vi "Auto_guider_queued.vi"() -> ()   [LabVIEW 2018]
uses:
  Global_Telescopio.vi
panel:
  out "respQ":refnum<queue>
  out "cmdQ":refnum<queue>
  in  "Case Constant\n(See Context Help) 2":bool
  in  "Case Constant\n(See Context Help)":bool=TRUE
  out "substring 3":string
  out "substring 2":string
  out "concatenated string":string
  out "substring":string
  out "result string":string
  in  "esc_placa":string="0.462"
  in  "guide_esp":string="S"
  in  "guide_cas":string="S"
  in  "guide_str":string="04/10/09  1:18:34\u000013 27 13\u0000-12 45 20\u0000"
  in  "guide_ang":string=" 281.52"
  in  "guide_nor":string="  11.53"
  in  "Tx_sts":u8[](array[numeric])=[22, 2, 1, 0, 83, 0, 0]
  out "rxsts 3":bool
  in  "SYN | ETX":u8[](array[numeric])=[22, 3] format="%02.0f"
  in  "tel_sts2":u8[](array[numeric])=[0, 0, 0] format="%02.0f"
  in  "Tx_ena":u8[](array[numeric])=[22, 2, 1, 0, 72, 0, 0] format="%02.0f"
  out "tel_sts1":bool[](array[boolean])=[TRUE, TRUE, TRUE, TRUE, FALSE, FALSE, TRUE]
  out "guide_dec":dbl format="%07.2g"
  out "guide_dir_ns":string
  out "guide_asc":dbl format="%07.2g"
  out "guide_dir_we":string
  in  "SYN | ACK":u8[](array[numeric])=[22, 6] format="%02.0f"
  out "rxsts":bool
  in  "Tx_nak":u8[](array[numeric])=[22, 21]
  out "Data rx guider":string
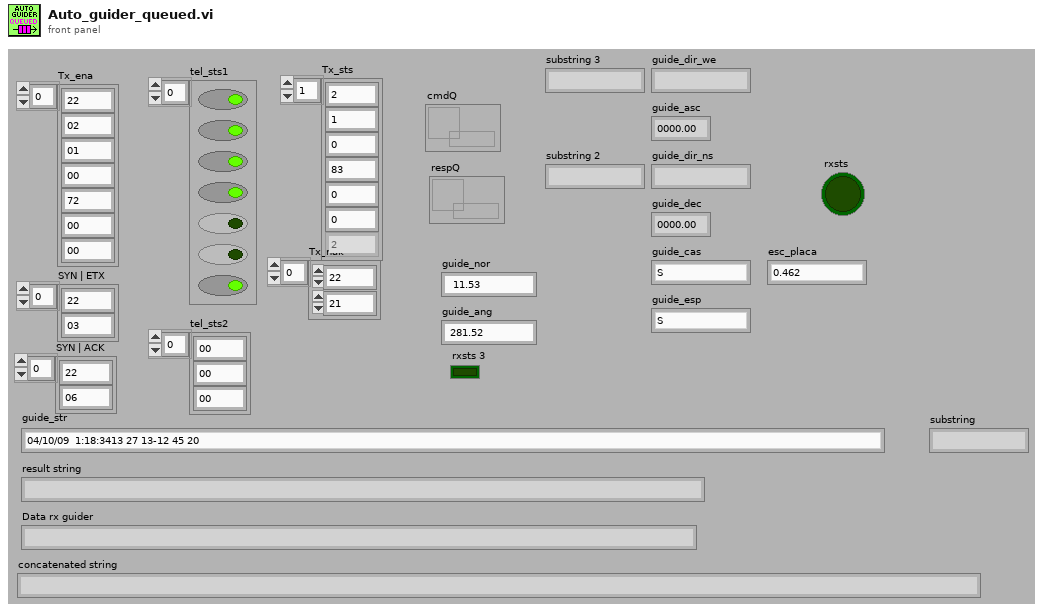
[diagram p1: front panel]
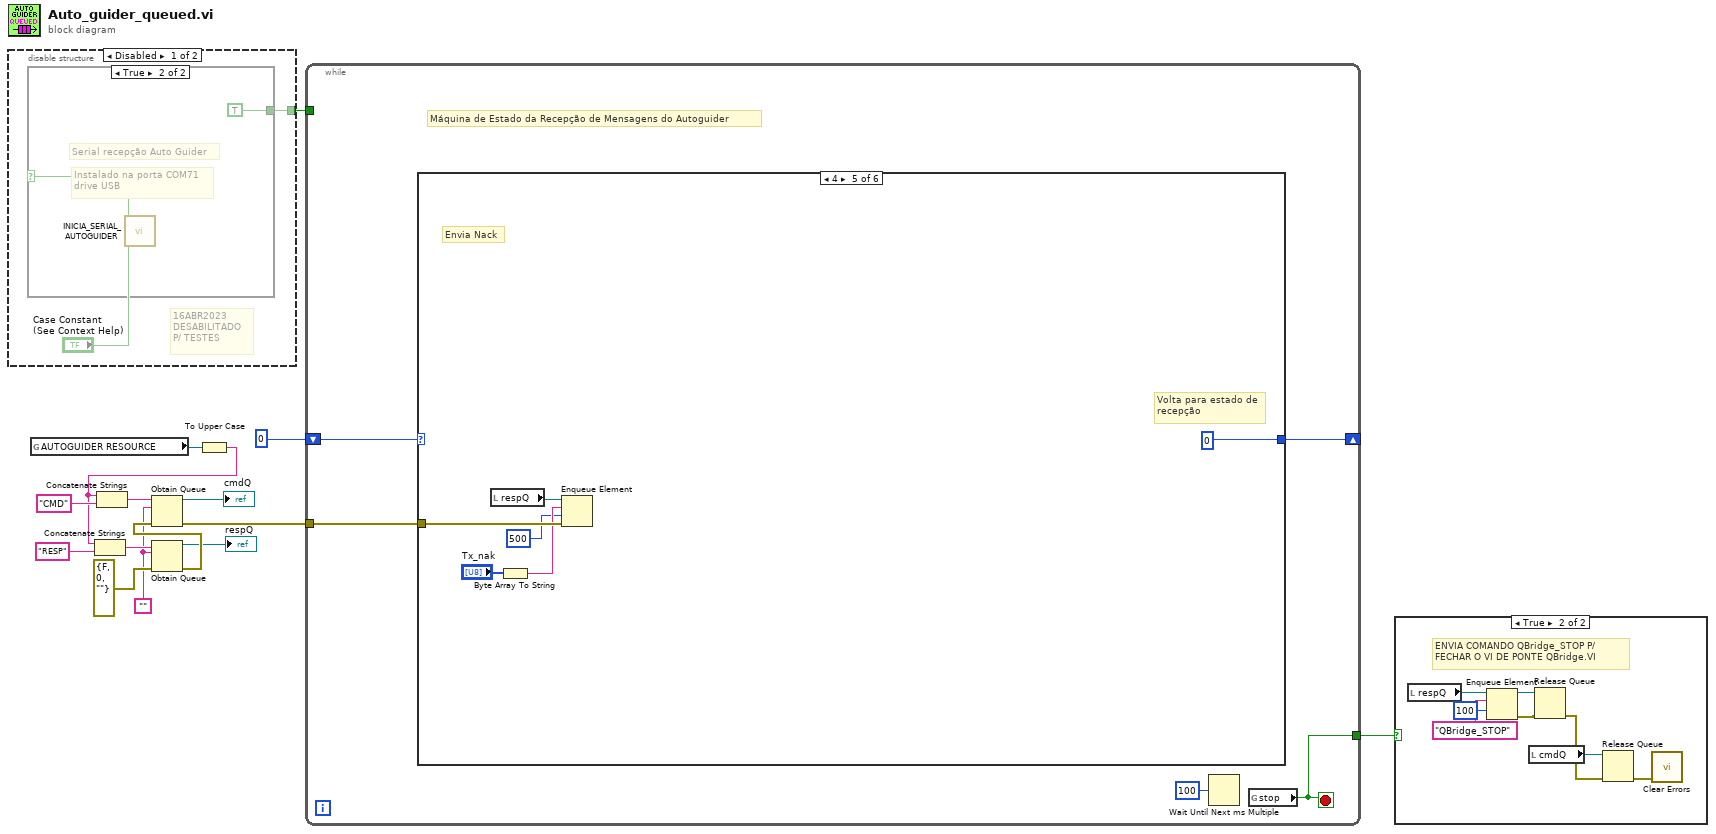
[diagram p0: block diagram]
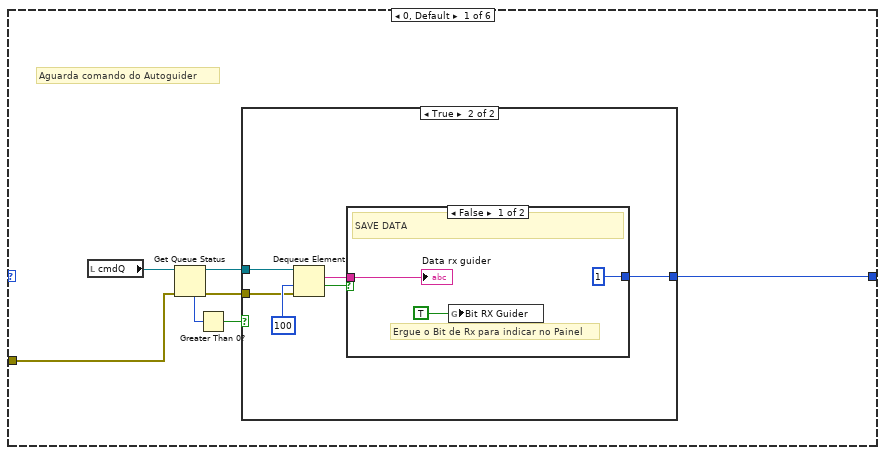
[diagram p5: hidden frame]
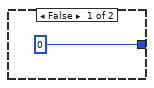
[diagram p6: hidden frame]
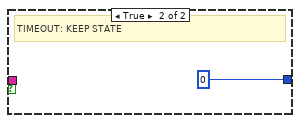
[diagram p7: hidden frame]
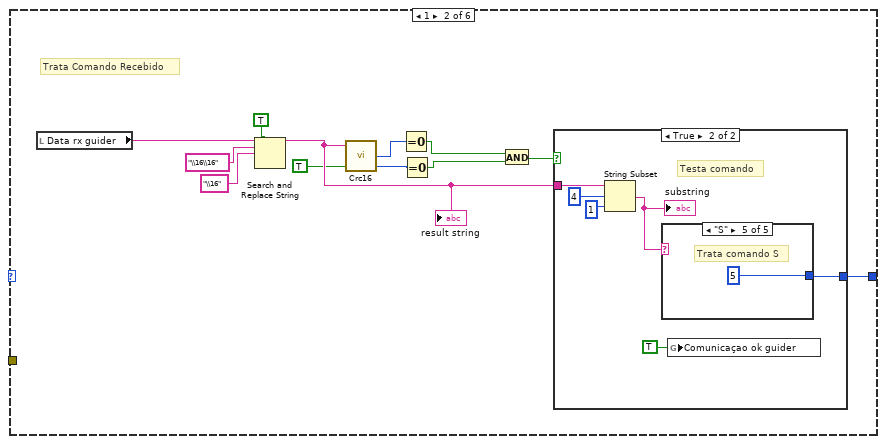
[diagram p8: hidden frame]
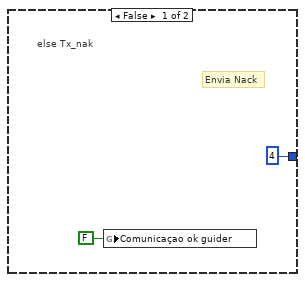
[diagram p9: hidden frame]
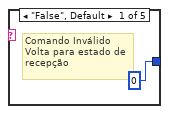
[diagram p10: hidden frame]
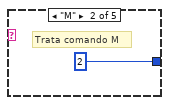
[diagram p11: hidden frame]
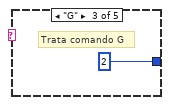
[diagram p12: hidden frame]
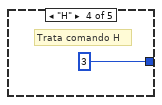
[diagram p13: hidden frame]
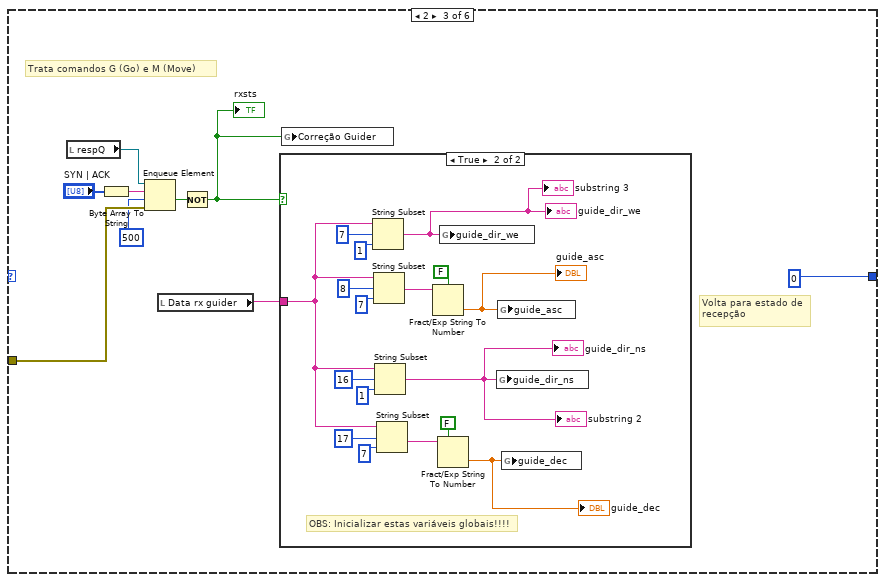
[diagram p14: hidden frame]
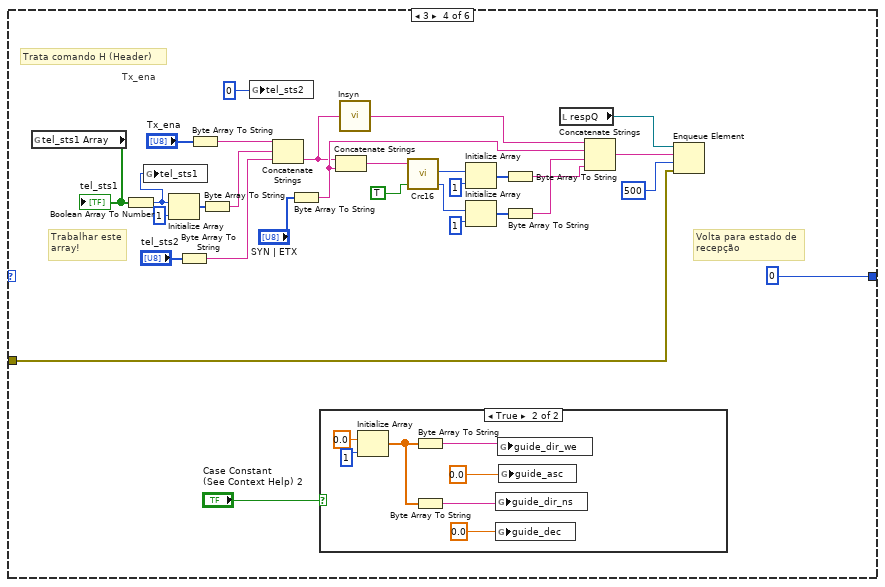
[diagram p16: hidden frame]
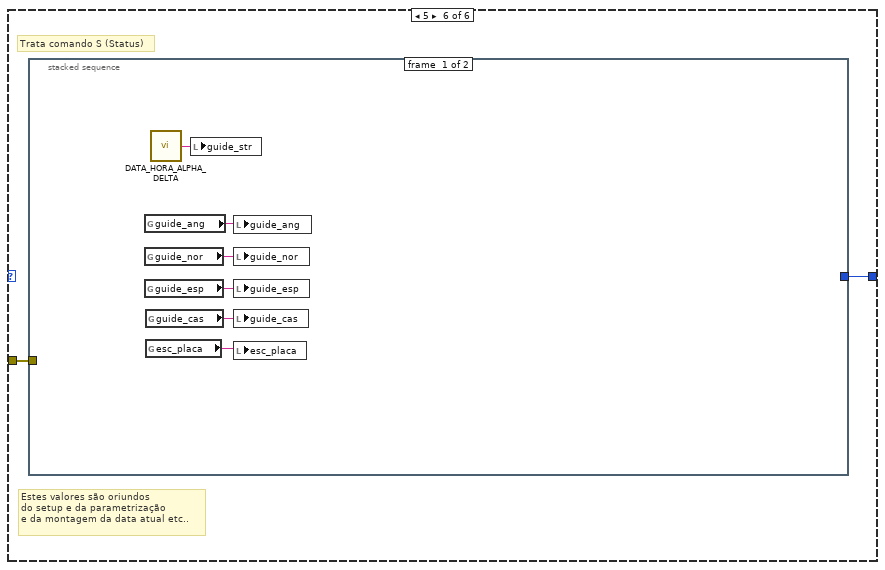
[diagram p18: hidden frame]
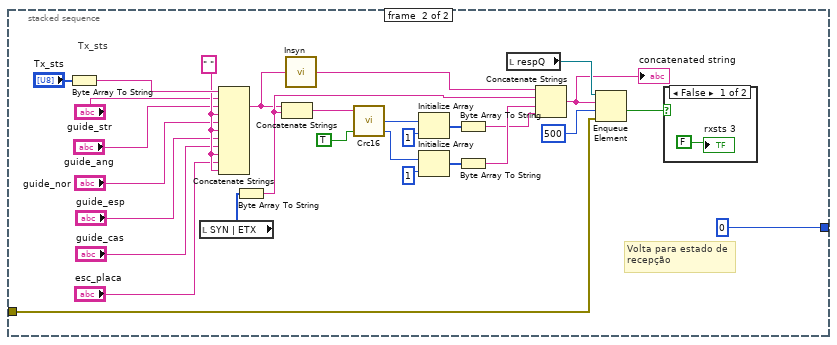
[diagram p19: hidden frame]
diagram:
  w2 = ""
  n1 = disable-structure shown="Disabled" {
    disable-tunnel: [w16 _] -> w14
    frame Disabled {
      # "16ABR2023\nDESABILITADO\nP/ TESTES"
      n2 = case shown="True" "Case Constant\n(See Context Help)" {
        tunnel: [_ TRUE] -> w16
        frame False {
        }
        frame True {
          # "Instalado na porta COM71\ndrive USB"
          # "Serial recepção Auto Guider"
          n3 = call "INICIA_SERIAL_AUTOGUIDER.vi"() -> ()  [unwired: 6 in, 1 out]
        }
      }
    }
    frame Enabled {
    }
  }
  n4 = global read "Global_Telescopio.vi" "AUTOGUIDER RESOURCE"() -> (w13:refnum<visa-resource-name>)
  n5 = To Upper Case(1:w13) -> (0:w10:string)
  n6 = Concatenate Strings(w10, "RESP" ("string")) -> (w9:string)
  n7 = Concatenate Strings(w10, "CMD" ("string")) -> (w8:string)
  n8 = Obtain Queue(name (unnamed)=w9, element data type=w2, error in (no error)=errorcluster {"status"=FALSE, "code"=0, "source"=""}) -> (queue out=→"respQ":refnum<queue>, error out=w6:errorcluster)  [unwired: 2 in, 1 out]
  n9 = Obtain Queue(name (unnamed)=w8, element data type=w2, error in (no error)=w6) -> (queue out=→"cmdQ":refnum<queue>, error out=w5:errorcluster)  [unwired: 2 in, 1 out]
  n10 = while {
    shift-right: [w21] -> _
    shift-left: 0 -> [w22]
    tunnel: w14 -> [_]
    tunnel: w5 -> [w20]
    tunnel: [w19] -> w1
    stop <- w19 stop-if-true
    # "Máquina de Estado da Recepção de Mensagens do Autoguider"
    n11 = case shown="4" w22 {
      tunnel: [w29 w53 0 0 0 w137] -> w21
      tunnel: w20 -> [w25 _ w71 w93 w132 w136]
      frame 0, Default {
        # "Aguarda comando do Autoguider"
        n12 = local read "cmdQ"() -> (w24:refnum<queue>)
        n13 = Get Queue Status(queue=w24, error in (no error)=w25) -> (queue out=w28:refnum<queue>, error out=w27:errorcluster, # elements in queue=w26:i32)  [unwired: 1 in, 5 out]
        n14 = Greater Than 0?(x=w26) -> (x > 0?=w30:bool)
        n15 = case shown="True" w30 {
          tunnel: [0 w37] -> w29
          tunnel: w27 -> [_ w33]
          tunnel: w28 -> [_ w32]
          frame False {
          }
          frame True {
            n16 = Dequeue Element(queue=w32, timeout in ms (-1)=100, error in (no error)=w33) -> (element=w35:string, timed out?=w36:bool)  [unwired: 2 out]
            n17 = case shown="False" w36 {
              tunnel: [1 0] -> w37
              tunnel: w35 -> [w38 _]
              frame False {
                # "Ergue o Bit de Rx para indicar no Painel"
                # "SAVE DATA"
                n18 = global write "Global_Telescopio.vi" "Bit RX Guider"(TRUE) -> ()
                "Data rx guider" <- w38
              }
              frame True {
                # "TIMEOUT: KEEP STATE"
              }
            }
          }
        }
      }
      frame 1 {
        # "Trata Comando Recebido"
        n19 = local read "Data rx guider"() -> (w49:string)
        n20 = Search and Replace String(replace all?=TRUE ("replace all? (F)"), input string=w49, search string="\\16\\16", replace string="\\16" ("replace string (\"\")")) -> (result string=w48:string)  [unwired: 4 in, 3 out]
        "result string" <- w48
        n21 = call "Crc16.vi"("Habilita"=TRUE, "tx_rx_buf"=w48) -> ("crc_lo"=w45:u8, "crc_hi"=w46:u8)  [unwired: 1 in, 1 out]
        n22 = Equal To 0?(x=w46) -> (x = 0?=w42:bool)
        n23 = Equal To 0?(x=w45) -> (x = 0?=w43:bool)
        n24 = And(x=w42, y=w43) -> (x .and. y?=w44:bool)
        n25 = case shown="True" w44 {
          tunnel: [4 w61] -> w53
          tunnel: w48 -> [_ w60]
          frame False {
            # "else Tx_nak"
            # "Envia Nack"
            n26 = global write "Global_Telescopio.vi" "Comunicaçao ok guider"(FALSE ("Comunicaçao ok guider")) -> ()
          }
          frame True {
            # "Testa comando"
            n27 = String Subset(string=w60, offset (0)=4, length (rest)=1 ("length (rest)")) -> (substring=w57:string)
            "substring" <- w57
            n28 = case shown="\"S\"" w57 {
              tunnel: [0 2 2 3 5] -> w61
              frame "False", Default {
                # "Comando Inválido\nVolta para estado de\nrecepção"
              }
              frame "M" {
                # "Trata comando M"
              }
              frame "G" {
                # "Trata comando G"
              }
              frame "H" {
                # "Trata comando H"
              }
              frame "S" {
                # "Trata comando S"
              }
            }
            n29 = global write "Global_Telescopio.vi" "Comunicaçao ok guider"(TRUE ("Comunicaçao ok guider")) -> ()
          }
        }
      }
      frame 2 {
        # "Volta para estado de\nrecepção"
        # "Trata comandos G (Go) e M (Move)"
        n30 = local read "respQ"() -> (w72:refnum<queue>)
        n31 = Byte Array To String(unsigned byte array="SYN | ACK") -> (string=w73:string)
        n32 = Enqueue Element(queue=w72, element=w73, timeout in ms (-1)=500, error in (no error)=w71) -> (timed out?=w69:bool)  [unwired: 2 out]
        n33 = local read "Data rx guider"() -> (w74:string)
        n34 = Not(x=w69) -> (.not. x?=w68:bool)
        "rxsts" <- w68
        n35 = case shown="True" w68 {
          tunnel: w74 -> [_ w88]
          frame False {
          }
          frame True {
            # "OBS: Inicializar estas variáveis globais!!!!"
            n36 = String Subset(string=w88, offset (0)=7, length (rest)=1 ("length (rest)")) -> (substring=w79:string)
            "guide_dir_we" <- w79
            "substring 3" <- w79
            n37 = String Subset(string=w88, offset (0)=8, length (rest)=7 ("length (rest)")) -> (substring=w83:string)
            n38 = String Subset(string=w88, offset (0)=16, length (rest)=1 ("length (rest)")) -> (substring=w77:string)
            "guide_dir_ns" <- w77
            "substring 2" <- w77
            n39 = String Subset(string=w88, offset (0)=17, length (rest)=7 ("length (rest)")) -> (substring=w82:string)
            n40 = Fract/Exp String To Number(use system decimal point (T)=FALSE, string=w83) -> (number=w78:dbl)  [unwired: 2 in, 1 out]
            "guide_asc" <- w78
            n41 = Fract/Exp String To Number(use system decimal point (T)=FALSE, string=w82) -> (number=w76:dbl)  [unwired: 2 in, 1 out]
            "guide_dec" <- w76
            n42 = global write "Global_Telescopio.vi" "guide_dir_we"(w79) -> ()
            n43 = global write "Global_Telescopio.vi" "guide_dir_ns"(w77) -> ()
            n44 = global write "Global_Telescopio.vi" "guide_asc"(w78) -> ()
            n45 = global write "Global_Telescopio.vi" "guide_dec"(w76) -> ()
          }
        }
        n46 = global write "Global_Telescopio.vi" "Correção Guider"(w68) -> ()
      }
      frame 3 {
        # "Volta para estado de\nrecepção"
        # "Trabalhar este\narray!"
        # "Tx_ena"
        # "Trata comando H (Header)"
        n47 = global read "Global_Telescopio.vi" "tel_sts1 Array"() -> (w99:bool[])
        "tel_sts1" <- w99
        n48 = Boolean Array To Number(Boolean array=w99) -> (number=w100:u32)
        n49 = global write "Global_Telescopio.vi" "tel_sts1"(w100) -> ()
        n50 = Initialize Array(w100, 1 ("dimension size")) -> (w107:u32[])
        n51 = Byte Array To String(unsigned byte array="tel_sts2") -> (string=w120:string)
        n52 = Byte Array To String(unsigned byte array="Tx_ena") -> (string=w118:string)
        n53 = Byte Array To String(unsigned byte array=w107) -> (string=w108:string)
        n54 = global write "Global_Telescopio.vi" "tel_sts2"(0) -> ()
        n55 = Concatenate Strings(w118, w108, w120) -> (w104:string)
        n56 = Byte Array To String(unsigned byte array="SYN | ETX") -> (string=w122:string)
        n57 = case shown="True" "Case Constant\n(See Context Help) 2" {
          frame False {
          }
          frame True {
            n58 = Initialize Array(0.0 ("element"), 1 ("dimension size")) -> (w127:dbl[])
            n59 = Byte Array To String(unsigned byte array=w127) -> (string=w126:string)
            n60 = Byte Array To String(unsigned byte array=w127) -> (string=w124:string)
            n61 = global write "Global_Telescopio.vi" "guide_dir_ns"(w124) -> ()
            n62 = global write "Global_Telescopio.vi" "guide_dec"(0.0 ("guide_dec")) -> ()
            n63 = global write "Global_Telescopio.vi" "guide_dir_we"(w126) -> ()
            n64 = global write "Global_Telescopio.vi" "guide_asc"(0.0 ("guide_asc")) -> ()
          }
        }
        n65 = Concatenate Strings(w104, w122) -> (w103:string)
        n66 = call "Insyn.vi"("txbuf"=w104) -> ("txbuf OUT"=w105:string)
        n67 = call "Crc16.vi"("Habilita"=TRUE, "tx_rx_buf"=w103) -> ("crc_lo"=w112:u8, "crc_hi"=w110:u8)  [unwired: 1 in, 1 out]
        n68 = Initialize Array(w110, 1 ("dimension size")) -> (w114:u8[])
        n69 = Initialize Array(w112, 1 ("dimension size")) -> (w113:u8[])
        n70 = Byte Array To String(unsigned byte array=w114) -> (string=w115:string)
        n71 = Byte Array To String(unsigned byte array=w113) -> (string=w116:string)
        n72 = local read "respQ"() -> (w96:refnum<queue>)
        n73 = Concatenate Strings(w105, w122, w116, w115) -> (w95:string)
        n74 = Enqueue Element(queue=w96, element=w95, timeout in ms (-1)=500, error in (no error)=w93) -> ()  [unwired: 3 out]
      }
      frame 4 {
        # "Volta para estado de\nrecepção"
        # "Envia Nack"
        n75 = local read "respQ"() -> (w133:refnum<queue>)
        n76 = Byte Array To String(unsigned byte array="Tx_nak") -> (string=w131:string)
        n77 = Enqueue Element(queue=w133, element=w131, timeout in ms (-1)=500, error in (no error)=w132) -> ()  [unwired: 3 out]
      }
      frame 5 {
        # "Estes valores são oriundos\ndo setup e da parametrização\ne da montagem da data atual etc.."
        # "Trata comando S (Status)"
        n78 = stacked-sequence {
          tunnel: [_ 0] -> w137
          tunnel: w136 -> [_ w147]
          frame #0 {
            n79 = global read "Global_Telescopio.vi" "guide_ang"() -> (w142:string)
            n80 = global read "Global_Telescopio.vi" "guide_nor"() -> (w141:string)
            n81 = global read "Global_Telescopio.vi" "guide_esp"() -> (w140:string)
            n82 = global read "Global_Telescopio.vi" "guide_cas"() -> (w139:string)
            n83 = global read "Global_Telescopio.vi" "esc_placa"() -> (w138:string)
            n84 = call "DATA_HORA_ALPHA_DELTA.vi"() -> ("SAIDA"=w143:string)  [unwired: 2 in]
            n85 = local write "guide_str"(w143) -> ()
            n86 = local write "guide_ang"(w142) -> ()
            n87 = local write "guide_nor"(w141) -> ()
            n88 = local write "guide_esp"(w140) -> ()
            n89 = local write "guide_cas"(w139) -> ()
            n90 = local write "esc_placa"(w138) -> ()
          }
          frame #1 {
            w161 = " " ("string")
            # "Volta para estado de\nrecepção"
            # "Tx_sts"
            n91 = Byte Array To String(unsigned byte array="Tx_sts") -> (string=w172:string)
            n92 = local read "SYN | ETX"() -> (w151:u8[])
            n93 = Concatenate Strings(w172, "guide_str", "guide_ang", w161, "guide_nor", w161, "guide_esp", "guide_cas", w161, "esc_placa", w161) -> (w159:string)
            n94 = Byte Array To String(unsigned byte array=w151) -> (string=w170:string)
            n95 = Concatenate Strings(w159, w170) -> (w158:string)
            n96 = call "Insyn.vi"("txbuf"=w159) -> ("txbuf OUT"=w160:string)
            n97 = call "Crc16.vi"("Habilita"=TRUE, "tx_rx_buf"=w158) -> ("crc_lo"=w166:u8, "crc_hi"=w167:u8)  [unwired: 1 in, 1 out]
            n98 = Initialize Array(w167, 1 ("dimension size")) -> (w165:u8[])
            n99 = Initialize Array(w166, 1 ("dimension size")) -> (w164:u8[])
            n100 = Byte Array To String(unsigned byte array=w165) -> (string=w168:string)
            n101 = Byte Array To String(unsigned byte array=w164) -> (string=w169:string)
            n102 = local read "respQ"() -> (w149:refnum<queue>)
            n103 = Concatenate Strings(w160, w170, w169, w168) -> (w148:string)
            "concatenated string" <- w148
            n104 = Enqueue Element(queue=w149, element=w148, timeout in ms (-1)=500, error in (no error)=w147) -> (timed out?=w144:bool)  [unwired: 2 out]
            n105 = case shown="False" w144 {
              frame False {
                "rxsts 3" <- FALSE ("rxsts")
              }
              frame True {
              }
            }
          }
        }
      }
    }
    n106 = Wait Until Next ms Multiple(millisecond multiple=u32 100) -> ()  [unwired: 1 out]
    n107 = global read "Global_Telescopio.vi" "stop"() -> (w19:bool)
  }
  n108 = case shown="True" w1 {
    frame False {
    }
    frame True {
      # "ENVIA COMANDO QBridge_STOP P/\nFECHAR O VI DE PONTE QBridge.VI"
      n109 = local read "respQ"() -> (w181:refnum<queue>)
      n110 = Enqueue Element(queue=w181, element="QBridge_STOP" ("x"), timeout in ms (-1)=100) -> (queue out=w179:refnum<queue>, error out=w177:errorcluster)  [unwired: 1 in, 1 out]
      n111 = local read "cmdQ"() -> (w180:refnum<queue>)
      n112 = Release Queue(queue=w179, error in (no error)=w177) -> (error out=w176:errorcluster)  [unwired: 1 in, 2 out]
      n113 = Release Queue(queue=w180, error in (no error)=w176) -> (error out=w175:errorcluster)  [unwired: 1 in, 2 out]
      n114 = call <vilib>:"Clear Errors.vi"("error in (no error)"=w175) -> ()  [unwired: 5 in, 2 out]
    }
  }
